vi "Get DUT Station Info.vi"(8 "error in (no error)":errorcluster, 10 "parameters in":T1, 11 "Sequencer Module runtime in":refnum<class "Sequencer Module runtime.lvclass">) -> (0 "error out":errorcluster, 1 "DUT Info out":T3, 2 "parameters out":T1, 3 "Sequencer Module runtime out":refnum<class "Sequencer Module runtime.lvclass">, 4 "Station Info out":T2)   [LabVIEW 2015, in "Sequencer Module runtime.lvclass"]
uses:
  Sequencer Module runtime.lvclass
  classes/Report Information/DUT Information.ctl
  classes/Report Information/Station Information.ctl
  <vilib>/NI/Tag Bus/table/data table.ctl
  Sequencer Module runtime.lvclass/Sequencer Module runtime.ctl
  <vilib>/NI/Tag Bus/table/data polymorphs/read one/read String.vi
  classes/Report Information/Report Information.lvclass
  <vilib>/NI/Tag Bus/table/data table.lvlib
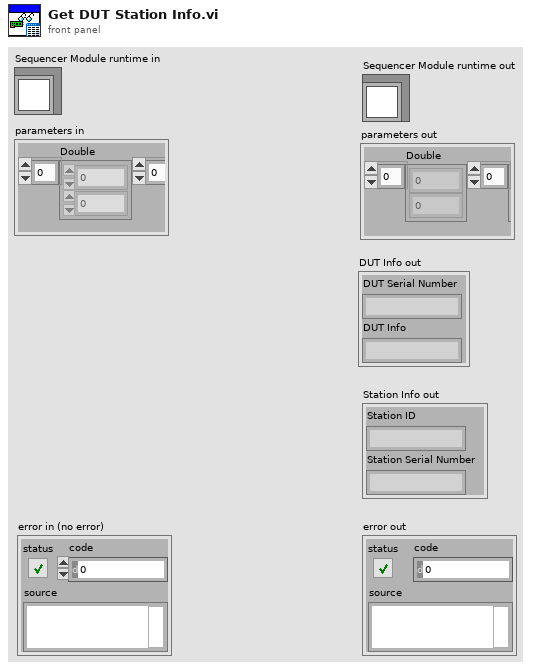
[diagram p1: front panel]
types:
  T1 = typedef "tag bus.lvlib/data table.lvlib/data table.ctl" = cluster{"Double":dbl[], "Single":sgl[], "I64":i64[], "I32":i32[], "I16":i16[], "I8":i8[], "U64":u64[], "U32":u32[], "U16":u16[], "U8":u8[], "Boolean":bool[], "String":string[], "Array of Double":cluster{"DBL Array":dbl[]}[], "Array of Single":cluster{"SGL Array":sgl[]}[], "Array of I64":cluster{"I64 Array":i64[]}[], "Array of I32":cluster{"I32 Array":i32[]}[], "Array of I16":cluster{"I16 Array":i16[]}[], "Array of I8":cluster{"I8 Array":i8[]}[], "Array of U64":cluster{"U64 Array":u64[]}[], "Array of U32":cluster{"U32 Array":u32[]}[], "Array of U16":cluster{"U16 Array":u16[]}[], "Array of U8":cluster{"U8 Array":u8[]}[], "Array of Boolean":cluster{"Boolean Array":bool[]}[], "Array of String":cluster{"String Array":string[]}[]}
  T2 = typedef "Report Information.lvclass/Station Information.ctl" = cluster{"Station ID":string, "Station Serial Number":string}
  T3 = typedef "Report Information.lvclass/DUT Information.ctl" = cluster{"DUT Serial Number":string, "DUT Info":string}
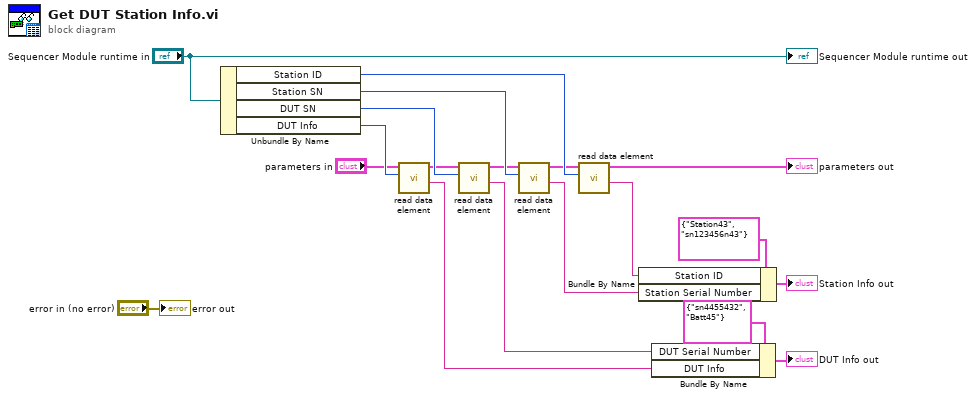
[diagram p0: block diagram]
diagram:
  n1 = Unbundle By Name("Sequencer Module runtime in") -> ("Station ID"=w15:i32, "Station SN"=w14:i32, "DUT SN"=w13:i32, "DUT Info"=w12:i32)
  n2 = call-poly <vilib>:"read data element.vi"("index"=w12, "data table in"="parameters in") -> ("value"=w2:string, "data table out"=w9:T1)  [unwired: 8 in]
  n3 = call-poly <vilib>:"read data element.vi"("index"=w13, "data table in"=w9) -> ("value"=w1:string, "data table out"=w8:T1)  [unwired: 8 in]
  n4 = call-poly <vilib>:"read data element.vi"("index"=w14, "data table in"=w8) -> ("value"=w3:string, "data table out"=w7:T1)  [unwired: 8 in]
  n5 = call-poly <vilib>:"read data element.vi"("index"=w15, "data table in"=w7) -> ("value"=w4:string, "data table out"=→"parameters out":T1)  [unwired: 8 in]
  n6 = Bundle By Name(cluster=T2 {"Station ID"="Station43", "Station Serial Number"="sn123456n43"} ("Station Info in"), "Station ID"=w4, "Station Serial Number"=w3) -> (→"Station Info out":T2)
  n7 = Bundle By Name(cluster=T3 {"DUT Serial Number"="sn4455432", "DUT Info"="Batt45"} ("DUT Info in"), "DUT Serial Number"=w1, "DUT Info"=w2) -> (→"DUT Info out":T3)
  "error out" <- "error in (no error)"
  "Sequencer Module runtime out" <- "Sequencer Module runtime in"
